vi "Queue Comms Dequeue.vi"(8 "error in (no error)":errorcluster) -> (0 "error out":errorcluster, 3 "element":T1)   [LabVIEW 2018, in "Testing UI 1.lvlib"]
doc: "This subVI dequeues an element from the communications queue using the Queue Comms FGV"
uses:
  Testing UI 1.lvlib
  Private Controls/Module Data.ctl
  Private Controls/Module Action.ctl
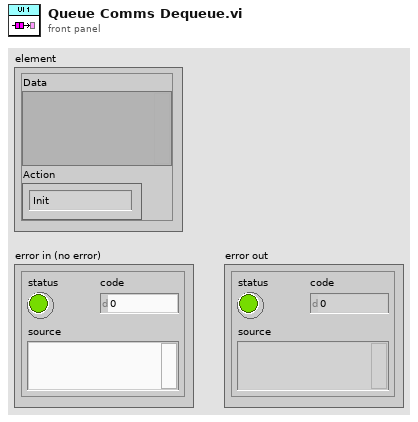
[diagram p1: front panel]
types:
  T1 = typedef "Testing UI 1.lvlib/Module Data.ctl" = cluster{"Data":variant, "Action":T2}
  T2 = typedef "Testing UI 1.lvlib/Module Action.ctl" = enum8{"Init", "Open FP", "Timeout", "New Report Value", "Update Test Info", "Record Data", "Update Report Path", "SetFuelPressure", "Error", "Exit", "Update System Log", "Load APU Setup Data", "Threshold ALERT", "Engine Start Val Change", "Value to Record"}
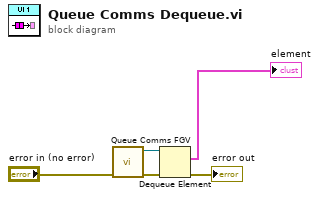
[diagram p0: block diagram]
diagram:
  n1 = call "Queue Comms FGV.vi"("error in (no error)"="error in (no error)") -> ("error out"=w4:errorcluster, "Queue out"=w3:refnum<queue>)  [unwired: 9 in]
  n2 = Dequeue Element(queue=w3, error in (no error)=w4) -> (element=→"element":T1, error out=→"error out":errorcluster)  [unwired: 1 in, 2 out]
